vi "User32dllAPI.ScreenSize.vi"() -> (0 "height":i16, 1 "width":i16)   [LabVIEW 2010]
uses:
  user32.dll
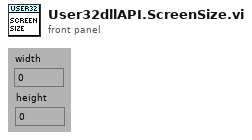
[diagram p1: front panel]
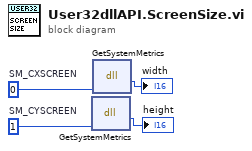
[diagram p0: block diagram]
diagram:
  w3 = 1  # SM_CYSCREEN
  w4 = 0  # SM_CXSCREEN
  n1 = dll-call lib="USER32.DLL" fn="GetSystemMetrics"("parameter"=w3) -> ("screenHeight"=→"height":i32)  [unwired: 4 in, 2 out]
  n2 = dll-call lib="USER32.DLL" fn="GetSystemMetrics"("parameter"=w4) -> ("screenWidth"=→"width":i32)  [unwired: 4 in, 2 out]
